vi "asdk Get Last Error.vi"(8 "error in (no error)":errorcluster, 10 "errSize":u32, 11 "errorNo":u32) -> (0 "error out":errorcluster, 2 "errMsg":string, 3 "errorNo out":u32)   [LabVIEW 2020, in "ASDK.lvlib"]
doc: "ASDK_API COMPL_STAT asdkGetLastError( UInt *errorNo, CString errMsg, Size_T errSize );"
uses:
  ASDK.lvlib
  ASDK.dll
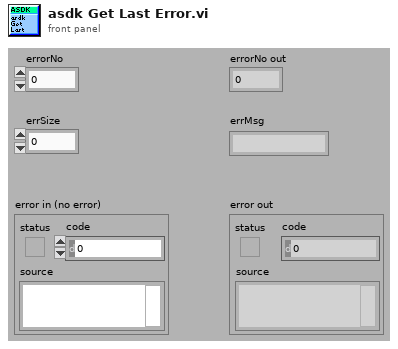
[diagram p1: front panel]
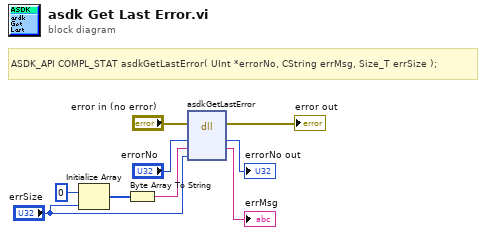
[diagram p0: block diagram]
diagram:
  # "ASDK_API COMPL_STAT asdkGetLastError( UInt *errorNo, CString errMsg, Size_T errSize );"
  n1 = Initialize Array(u8 0 ("element"), "errSize") -> (w7:u8[])
  n2 = Byte Array To String(unsigned byte array=w7) -> (string=w6:string)
  n3 = dll-call lib="ASDK.*" fn="asdkGetLastError"(error in="error in (no error)", "errorNo"="errorNo", "errMsg"=w6, "errSize"="errSize") -> (error out=→"error out":errorcluster, "errorNo"=→"errorNo out":u32, "errMsg"=→"errMsg":string)  [unwired: 4 in, 1 out]
